vi "FullProject.vi"() -> ()   [LabVIEW 2020]
uses:
  <vilib>/Instr/_visa.llb/VISA Configure Serial Port (Instr).vi
  <vilib>/picture/3D Picture Control/Object/Create Object (name).vi
  <vilib>/picture/3D Picture Control/Object/Add Object (no reference).vi
  <vilib>/picture/3D Picture Control/NI_3D Picture Control.lvlib
panel:
  out "East/West":string
  out "North/South":string
  out "ID":string
  out "Altitude":dbl
  out "Pos-Fix":dbl
  out "Satellite":dbl
  out "Longtitude":dbl
  out "Latitude":dbl
  out "UTC":dbl
  out "Pressure":dbl(knob) scale=0.0..2000.0
  out "theta":dbl
  out "epsi":dbl
  out "phi":dbl
  out "3D Picture":refnum<vi>(3d-picture)
  out "Humidity":dbl(knob) scale=0.0..100.0
  out "Thermometer":dbl(slide) scale=0.0..100.0
  in  "stop":bool
  out "read buffer":string
  in  "VISA resource name":refnum<visa-resource-name>
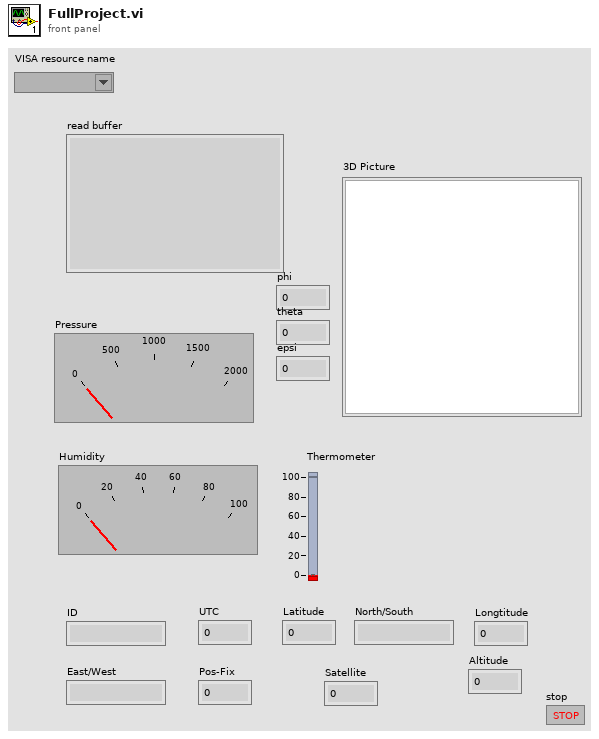
[diagram p1: front panel]
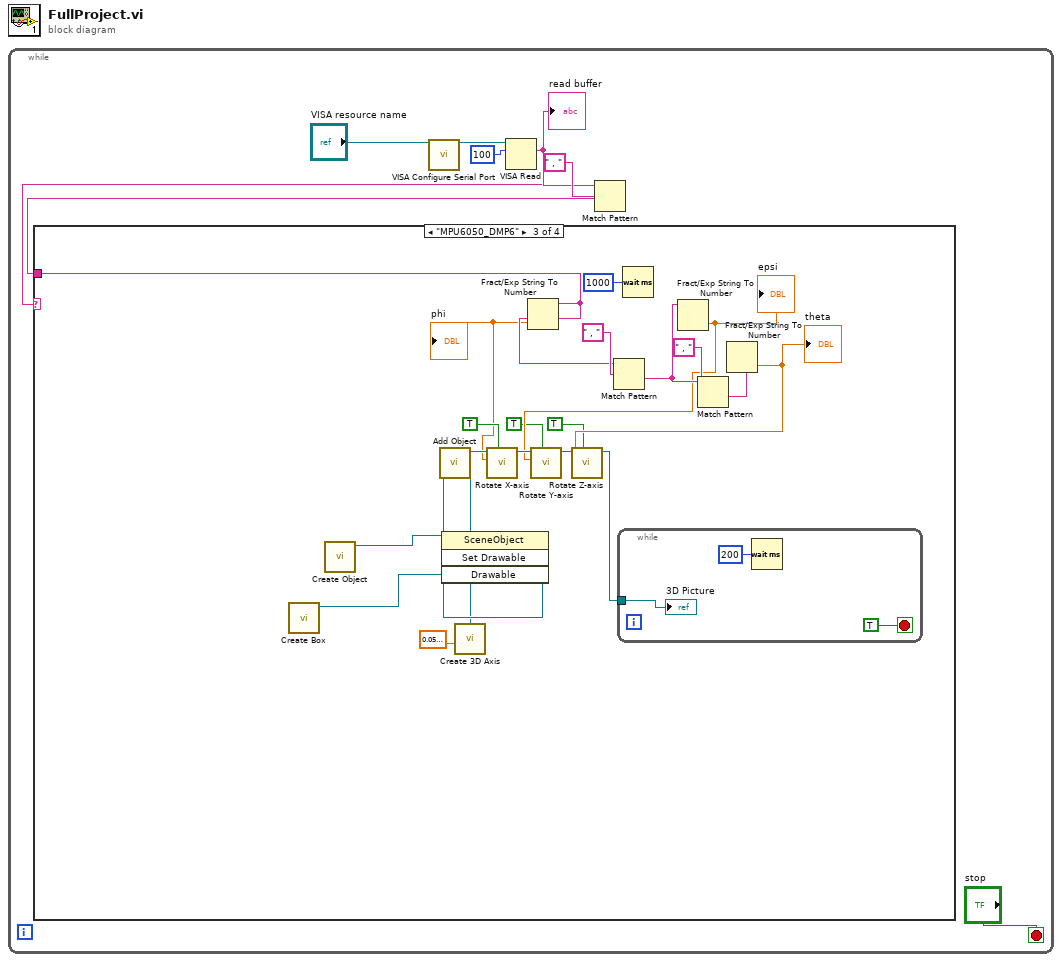
[diagram p0: block diagram]
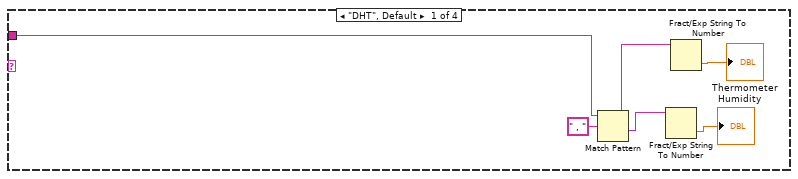
[diagram p2: hidden frame]
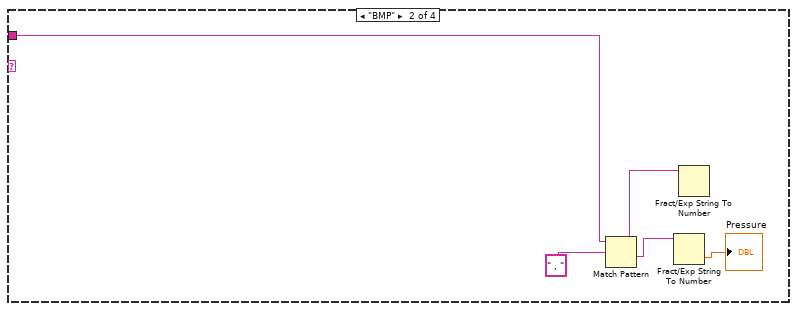
[diagram p3: hidden frame]
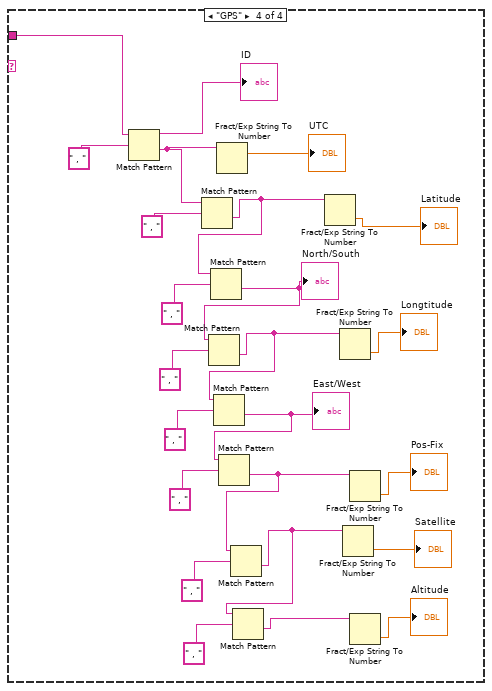
[diagram p4: hidden frame]
diagram:
  n1 = while {
    stop <- "stop" stop-if-true
    n2 = call-poly "VISA Configure Serial Port"("VISA resource name"="VISA resource name") -> ("VISA resource name out"=w7:refnum<visa-resource-name>)  [unwired: 13 in, 1 out]
    n3 = VISA Read(VISA resource name=w7, byte count=u32 100) -> (read buffer=w3:string)  [unwired: 1 in, 3 out]
    "read buffer" <- w3
    n4 = Match Pattern(string=w3, regular expression=" , ") -> (before substring=w2:string, after substring=w1:string)  [unwired: 1 in, 2 out]
    n5 = case shown="\"MPU6050_DMP6\"" w2 {
      tunnel: w1 -> [w10 w15 w36 w66]
      frame "DHT", Default {
        n6 = Match Pattern(string=w10, regular expression=" , ") -> (before substring=w9:string, after substring=w13:string)  [unwired: 1 in, 2 out]
        n7 = Fract/Exp String To Number(string=w13) -> (number=→"Humidity":dbl)  [unwired: 3 in, 1 out]
        n8 = Fract/Exp String To Number(string=w9) -> (number=→"Thermometer":dbl)  [unwired: 3 in, 1 out]
      }
      frame "BMP" {
        n9 = Match Pattern(string=w15, regular expression=" , ") -> (before substring=w16:string, after substring=w19:string)  [unwired: 1 in, 2 out]
        n10 = Fract/Exp String To Number(string=w19) -> (number=→"Pressure":dbl)  [unwired: 3 in, 1 out]
        n11 = Fract/Exp String To Number(string=w16) -> ()  [unwired: 3 in, 2 out]
      }
      frame "MPU6050_DMP6" {
        n12 = call <vilib>:"Create Box.vi"() -> ("New Box Refnum"=w20:refnum<vi>)  [unwired: 10 in, 1 out]
        n13 = call-poly <vilib>:"Create Object.vi"() -> ("Scene:New Object"=w35:refnum<vi>)  [unwired: 10 in, 1 out]
        n14 = invoke class="SceneObject" method="Set Drawable"(reference=w35, "Drawable"=w20) -> (reference out=w34:refnum<vi>)  [unwired: 2 in, 3 out]
        n15 = call <vilib>:"Create 3D Axis.vi"("Radius"=sgl 0.05) -> ("New Object Refnum"=w33:refnum<vi>)  [unwired: 9 in, 1 out]
        n16 = call-poly <vilib>:"Add Object.vi"("New Object In"=w33, "Scene Object In"=w34) -> ("Scene Object Out"=w31:refnum<vi>)  [unwired: 8 in, 1 out]
        n17 = Fract/Exp String To Number(string=w36) -> (number=w23:dbl)  [unwired: 3 in, 1 out]
        "phi" <- w23
        n18 = call <vilib>:"Rotate X-axis.vi"("Relative?"=TRUE, "angle"=w23, "Scene Object In"=w31) -> ("Scene Object Out"=w30:refnum<vi>)  [unwired: 7 in, 1 out]
        n19 = Match Pattern(string=w36, regular expression=" , ") -> (after substring=w40:string)  [unwired: 1 in, 3 out]
        n20 = Wait (ms)(milliseconds to wait=u32 1000) -> ()  [unwired: 1 out]
        n21 = Fract/Exp String To Number(string=w40) -> (number=w28:dbl)  [unwired: 3 in, 1 out]
        "epsi" <- w28
        n22 = call <vilib>:"Rotate Y-axis.vi"("Relative?"=TRUE, "angle"=w28, "Scene Object In"=w30) -> ("Scene Object Out"=w29:refnum<vi>)  [unwired: 7 in, 1 out]
        n23 = Match Pattern(string=w40, regular expression=" , ") -> (after substring=w39:string)  [unwired: 1 in, 3 out]
        n24 = Fract/Exp String To Number(string=w39) -> (number=w27:dbl)  [unwired: 3 in, 1 out]
        "theta" <- w27
        n25 = call <vilib>:"Rotate Z-axis.vi"("Relative?"=TRUE, "angle"=w27, "Scene Object In"=w29) -> ("Scene Object Out"=w22:refnum<vi>)  [unwired: 7 in, 1 out]
        n26 = while {
          tunnel: w22 -> [w42]
          stop <- TRUE stop-if-true
          n27 = Wait (ms)(milliseconds to wait=u32 200) -> ()  [unwired: 1 out]
          "3D Picture" <- w42
        }
      }
      frame "GPS" {
        n28 = Match Pattern(string=w66, regular expression=" , ") -> (before substring=→"ID":string, after substring=w58:string)  [unwired: 1 in, 2 out]
        n29 = Match Pattern(string=w58, regular expression=" , ") -> (after substring=w55:string)  [unwired: 1 in, 3 out]
        n30 = Match Pattern(string=w55, regular expression=" , ") -> (after substring=w53:string)  [unwired: 1 in, 3 out]
        "North/South" <- w53
        n31 = Match Pattern(string=w53, regular expression=" , ") -> (after substring=w48:string)  [unwired: 1 in, 3 out]
        n32 = Match Pattern(string=w48, regular expression=" , ") -> (after substring=w44:string)  [unwired: 1 in, 3 out]
        "East/West" <- w44
        n33 = Fract/Exp String To Number(string=w58) -> (number=→"UTC":dbl)  [unwired: 3 in, 1 out]
        n34 = Match Pattern(string=w44, regular expression=" , ") -> (after substring=w45:string)  [unwired: 1 in, 3 out]
        n35 = Match Pattern(string=w45, regular expression=" , ") -> (after substring=w46:string)  [unwired: 1 in, 3 out]
        n36 = Match Pattern(string=w46, regular expression=" , ") -> (after substring=w47:string)  [unwired: 1 in, 3 out]
        n37 = Fract/Exp String To Number(string=w55) -> (number=→"Latitude":dbl)  [unwired: 3 in, 1 out]
        n38 = Fract/Exp String To Number(string=w48) -> (number=→"Longtitude":dbl)  [unwired: 3 in, 1 out]
        n39 = Fract/Exp String To Number(string=w46) -> (number=→"Satellite":dbl)  [unwired: 3 in, 1 out]
        n40 = Fract/Exp String To Number(string=w45) -> (number=→"Pos-Fix":dbl)  [unwired: 3 in, 1 out]
        n41 = Fract/Exp String To Number(string=w47) -> (number=→"Altitude":dbl)  [unwired: 3 in, 1 out]
      }
    }
  }
